vi "FLOM Test Program.vi"() -> ()   [LabVIEW 2021, in "FLOM Pump.lvlib"]
uses:
  FLOM Pump.lvlib
  Settings Cluster.ctl
panel:
  in  "stop":bool
  out "Pressure":dbl
  out "Flow Rate":dbl
  out "Connection Error":bool
  out "No Pump Connected":bool
  out "Pump On?":enum16{"Off", "On", "Not Initialized"}(ring)
  in  "Speed":dbl
  in  "VICI Settings":T1={"VISA resource name"="COM4", "Simulated?"=FALSE, "Pump Number"=1.0}
  in  "Pause":bool
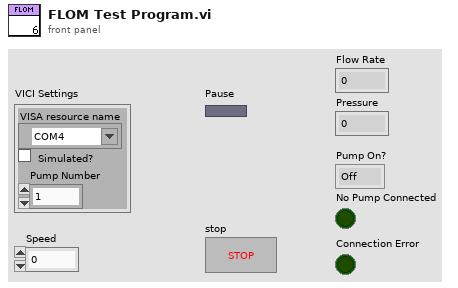
[diagram p1: front panel]
types:
  T1 = typedef "FLOM Pump.lvlib/Settings Cluster.ctl" = cluster{"VISA resource name":refnum<visa-resource-name>, "Simulated?":bool, "Pump Number":dbl}
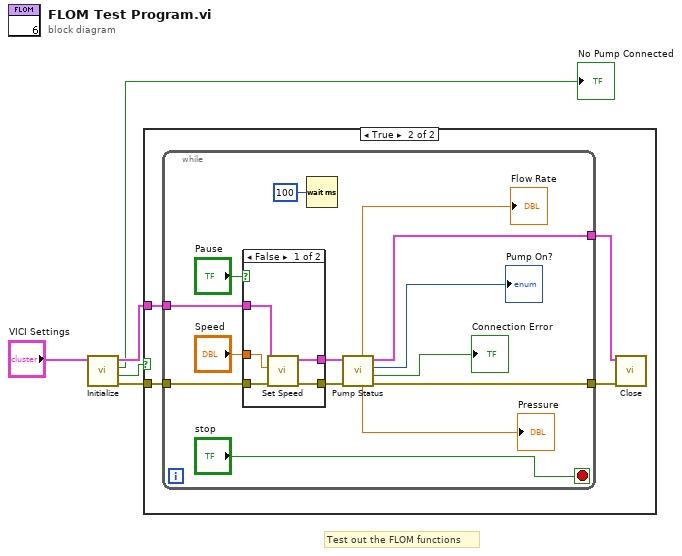
[diagram p0: block diagram]
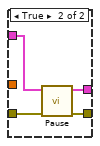
[diagram p3: hidden frame]
diagram:
  # "Test out the FLOM functions"
  n1 = call "Initialize.vi"("FLOM Settings in"="VICI Settings") -> ("error out"=w3:errorcluster, "Initialized"=w2:bool, "No Pump Connected"=→"No Pump Connected":bool, "FLOM Settings out"=w4:T1)  [unwired: 7 in]
  n2 = case shown="True" w2 {
    tunnel: w4 -> [_ w9]
    tunnel: w3 -> [_ w8]
    frame False {
    }
    frame True {
      n3 = while {
        tunnel: w9 -> [w22]
        tunnel: w8 -> [w21]
        tunnel: [w18] -> w7
        tunnel: [w17] -> w6
        stop <- "stop" stop-if-true
        n4 = case shown="False" "Pause" {
          tunnel: w22 -> [w28 w30]
          tunnel: w21 -> [w27 w29]
          tunnel: [w26 w31] -> w20
          tunnel: [w25 w32] -> w19
          tunnel: "Speed" -> [w24 _]
          frame False {
            n5 = call "Set Speed.vi"("error in (no error)"=w27, "speed"=w24, "FLOM Settings in"=w28) -> ("error out"=w26:errorcluster, "FLOM Settings out"=w25:T1)  [unwired: 6 in, 1 out]
          }
          frame True {
            n6 = call "Pause.vi"("error in (no error)"=w29, "FLOM Settings in"=w30) -> ("error out"=w31:errorcluster, "FLOM Settings out"=w32:T1)  [unwired: 7 in, 1 out]
          }
        }
        n7 = Wait (ms)(milliseconds to wait=u32 100) -> ()  [unwired: 1 out]
        n8 = call "Pump Status.vi"("error in (no error)"=w20, "FLOM Settings In"=w19) -> ("error out"=w17:errorcluster, "Connection Error"=→"Connection Error":bool, "Pump On?"=→"Pump On?":enum16{"Off", "On", "Not Initialized"}, "FLOM Settings Out"=w18:T1, "Pressure"=→"Pressure":dbl, "Flow Rate"=→"Flow Rate":dbl)  [unwired: 4 in]
      }
      n9 = call "Close.vi"("error in (no error)"=w6, "FLOM Settings in"=w7) -> ()  [unwired: 7 in, 3 out]
    }
  }
